vi "From String.vi"(8 "error in (no error)":errorcluster, 9 "initial scan location":u32, 10 "String":string, 11 "Type in":refnum<class "Abs_String.lvclass">) -> (0 "error out":errorcluster, 1 "offset past scan":u32, 2 "Remaining String":string, 3 "Type out":refnum<class "Abs_String.lvclass">)   [LabVIEW 2021, in "Abs_String.lvclass"]
uses:
  Abs_String.lvclass
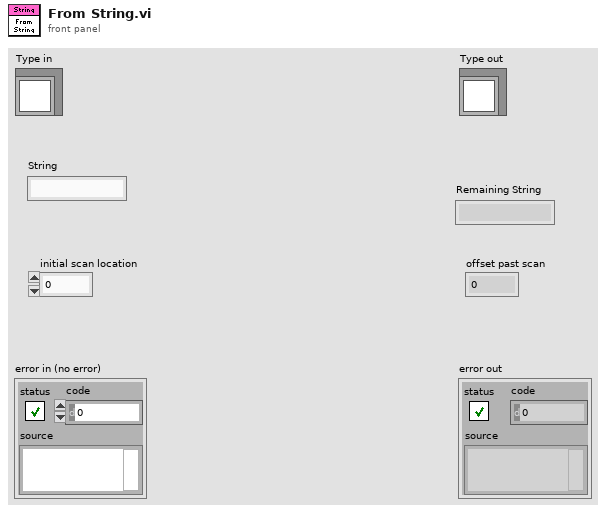
[diagram p1: front panel]
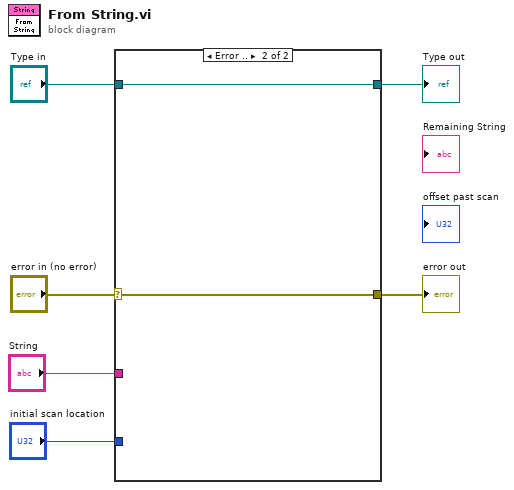
[diagram p0: block diagram]
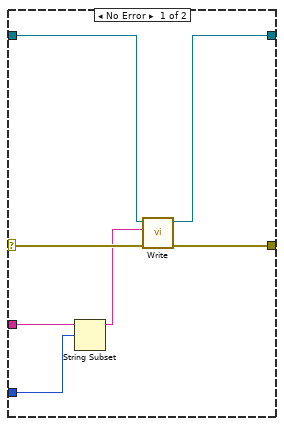
[diagram p2: hidden frame]
diagram:
  n1 = case shown="Error .." "error in (no error)" {
    selector: "error in (no error)" -> [w13 w15]
    tunnel: [w12 w15] -> w5
    tunnel: "Type in" -> [w11 w14]
    tunnel: [w10 w14] -> w3
    tunnel: "String" -> [w9 _]
    tunnel: "initial scan location" -> [w7 _]
    frame No Error {
      n2 = String Subset(string=w9, offset (0)=w7) -> (substring=w8:string)  [unwired: 1 in]
      n3 = call-dynamic "Write.vi"("error in (no error)"=w13, "String"=w8, "Abs_String in"=w11) -> ("error out"=w12:errorcluster, "Abs_String out"=w10:refnum<class "Abs_String.lvclass">)  [unwired: 7 in]
    }
    frame Error {
    }
  }
  "error out" <- w5
  "Type out" <- w3
